vi "niScope Multi Fetch Complex WDT.vi"(5 "timestamp Type":T1=1 caption="timestamp type" items=["relative", "absolute"], 7 "timeout":dbl=5.0 format="%.2f", 8 "error in":errorcluster, 9 "numSamples":i32=-1, 10 "channels":string="0", 11 "instrument handle":refnum<k15>) -> (0 "error out":errorcluster, 1 "wfm":waveform(cdb)[](array[waveform]), 2 "wfm info":T2(array[cluster]) {"reserved2" format="%.2f"; "reserved1" format="%.2f"; "offset" format="%^.3e"; "gain" format="%^.3e"; "xIncrement" format="%^.3e"; "relativeInitialX" format="%^.3e"; "absoluteInitialX" format="%^.3e"}, 3 "instrument handle out":refnum<k15>)   [LabVIEW 2011]
doc: "Retrieves complex waveforms the digitizer has acquired from multiple records or multiple channels. Returns a two-dimensional array of LabVIEW complex waveform data types that includes timing information."
uses:
  <instrlib>/niScope/Controls/niScope timestamp type.ctl
  niScope_32.dll
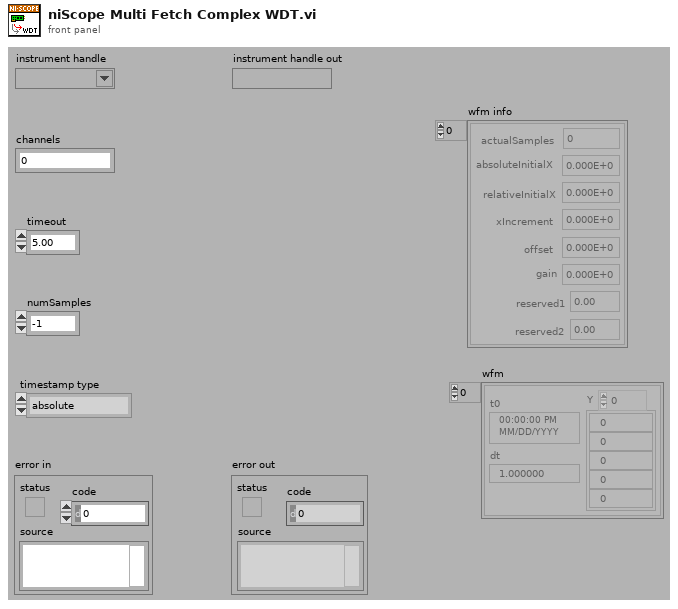
[diagram p1: front panel]
types:
  T1 = typedef "niScope timestamp type.ctl" = i32
  T2 = cluster{"actualSamples":i32, "absoluteInitialX":dbl, "relativeInitialX":dbl, "xIncrement":dbl, "offset":dbl, "gain":dbl, "reserved1":dbl, "reserved2":dbl}[]
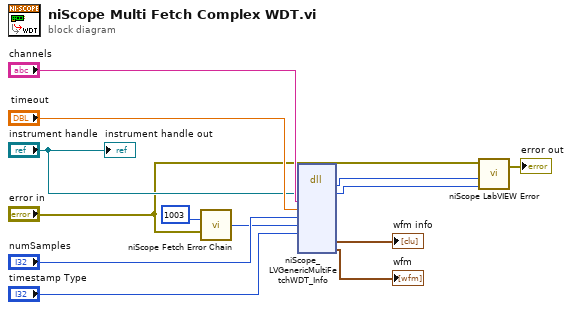
[diagram p0: block diagram]
diagram:
  n1 = call <instrlib>:"niScope Fetch Error Chain.vi"("dataType in"=1003 ("dataType"), "error in"="error in") -> ("dataType"=w4:i32)  [unwired: 13 in]
  n2 = dll-call lib="niScope_*.*" fn="niScope_LVGenericMultiFetchWDT_Info"("instrument handle"="instrument handle", "channelList"="channels", "timeout"="timeout", "numSamples"="numSamples", "dataType"=w4, "timestampType"="timestamp Type") -> ("status"=w9:i32, "instrument handle"=w8:u32, "wfm info"=→"wfm info":T2, "wfm"=→"wfm":waveform(cdb)[])  [unwired: 10 in, 2 out]
  n3 = call <instrlib>:"niScope LabVIEW Error.vi"("instrument handle"=w8, "niScope error code (0)"=w9, "error in (no error)"="error in") -> ("error out"=→"error out":errorcluster)  [unwired: 2 in]
  "instrument handle out" <- "instrument handle"
